vi "1.1 Friction Function.vi"(1 "Controls Output":fxp<+/-,20,5> format="%.17g", 2 "Input F":fxp<+/-,20,5> format="%.17g") -> (0 "Friction Modified Output":fxp<+/-,20,5> format="%.17g")   [LabVIEW 2011]
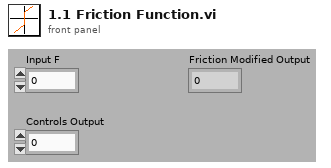
[diagram p1: front panel]
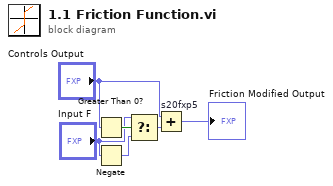
[diagram p0: block diagram]
diagram:
  n1 = Greater Than 0?(x="Controls Output") -> (x > 0?=w4:bool)
  n2 = Negate(x="Input F") -> (-x=w2:fxp<+/-,21,6>)
  n3 = Select(t="Input F", s=w4, f=w2) -> (s? t:f=w3:fxp<+/-,21,6>)
  n4 = Add "s20fxp5"(x="Controls Output", y=w3) -> (x+y=→"Friction Modified Output":fxp<+/-,20,5>)
